vi "FIXME#253_MAV_MSG_STATUSTEXT_ENCODE.vi"(10 "packet_sequence_in":u8, 11 "STATUSTEXT":T1={"severity"=enum."MAV_SEVERITY_INFO", "id"=0, "chunk_seq"=0, "text"="Labview Ground Control Station 0.1", "self"={"system_id"=255, "component_id"=190}}) -> (2 "packet_sequence_out":u8, 3 "mavlink_buffer_out":u8[](array[numeric]))   [LabVIEW 2023]
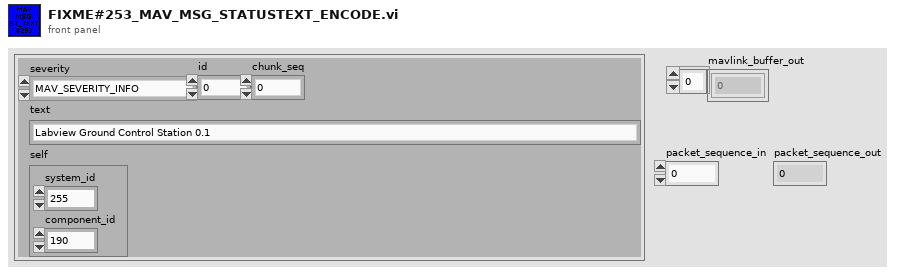
[diagram p1: front panel]
types:
  T1 = cluster{"severity":enum8{"MAV_SEVERITY_EMERGENCY", "MAV_SEVERITY_ALERT", "MAV_SEVERITY_CRITICAL", "MAV_SEVERITY_ERROR", "MAV_SEVERITY_WARNING", "MAV_SEVERITY_NOTICE", "MAV_SEVERITY_INFO", "MAV_SEVERITY_DEBUG"}, "id":u16, "chunk_seq":u8, "text":string, "self":cluster{"system_id":u8, "component_id":u8}}
  T2 = enum8{"MAV_SEVERITY_EMERGENCY", "MAV_SEVERITY_ALERT", "MAV_SEVERITY_CRITICAL", "MAV_SEVERITY_ERROR", "MAV_SEVERITY_WARNING", "MAV_SEVERITY_NOTICE", "MAV_SEVERITY_INFO", "MAV_SEVERITY_DEBUG"}
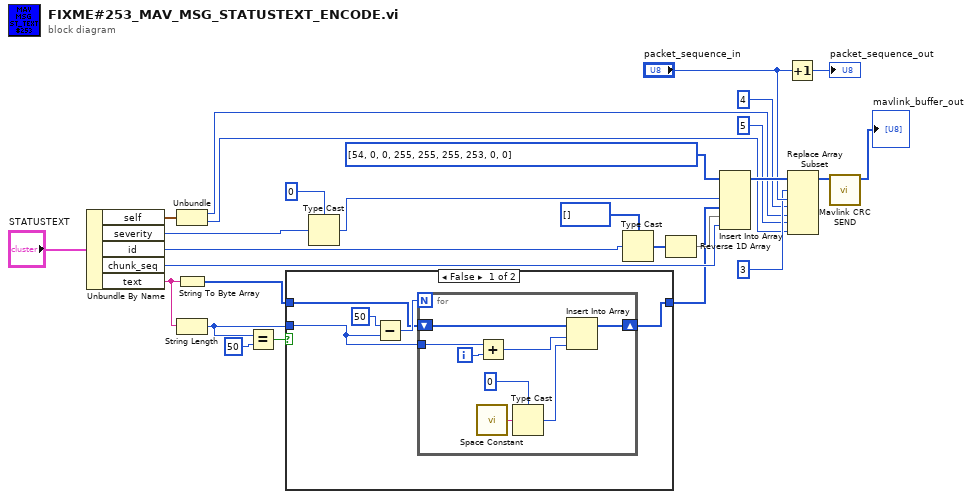
[diagram p0: block diagram]
diagram:
  n1 = Unbundle By Name("STATUSTEXT") -> ("self"=w23:cluster{"system_id":u8, "component_id":u8}, "severity"=w14:T2, "id"=w12:u16, "chunk_seq"=w8:u8, "text"=w2:string)
  n2 = Unbundle(w23) -> ("system_id"=w18:u8, "component_id"=w17:u8)
  n3 = String To Byte Array(string=w2) -> (unsigned byte array=w1:u8[])
  n4 = String Length(string=w2) -> (length=w4:i32)
  n5 = Equal?(x=w4, y=50) -> (x = y?=w5:bool)
  n6 = case shown="False" w5 {
    tunnel: [w29 w41] -> w3
    tunnel: w1 -> [w30 w41]
    tunnel: w4 -> [w28 _]
    frame False {
      n7 = Subtract(x=50, y=w28) -> (x-y=w31:i32)
      n8 = for {
        N: w31 -> [_]
        shift-right: [w40] -> w29
        shift-left: w30 -> [w39]
        tunnel: w28 -> [w37]
        i -> [w38]
        n9 = call <vilib>:"Space Constant.vi"() -> ("String"=w35:string)
        n10 = Add(x=w37, y=w38) -> (x+y=w36:i32)
        n11 = Type Cast(type=u8 0 ("new element/subarray"), x=w35) -> (*(type *) &x=w33:u8)
        n12 = Insert Into Array(array=w39, index=w36, new element=w33) -> (w40:u8[])
      }
    }
    frame True {
    }
  }
  n13 = Type Cast(type=u8 0 ("index"), x=w14) -> (*(type *) &x=w13:u8)
  n14 = Type Cast(type=u8[] [] ("index"), x=w12) -> (*(type *) &x=w10:u8[])
  n15 = Reverse 1D Array(array=w10) -> (reversed array=w9:u8[])
  n16 = Insert Into Array(array=u8[] [54, 0, 0, 255, 255, 255, 253, 0, 0], new element #1=w13, new element #2=w3, new element #3=w9, new element #4=w8) -> (w26:u8[])  [unwired: 1 in]
  n17 = Increment(x="packet_sequence_in") -> (x+1=→"packet_sequence_out":u8)
  n18 = Replace Array Subset(array=w26, new element #1="packet_sequence_in", index #1=3 ("index"), new element #2=w18, index #2=4 ("index"), new element #3=w17, index #3=5 ("index")) -> (w16:u8[])
  n19 = call "Mavlink CRC SEND.vi"("Byte In"=w16) -> ("Output Byte"=→"mavlink_buffer_out":u8[])  [unwired: 10 in]
